vi "setUp.vi"(8 "error in (no error)":errorcluster, 11 "reference in":refnum<class "RT Stop.lvclass">) -> (0 "error out":errorcluster, 3 "reference out":refnum<class "RT Stop.lvclass">)   [LabVIEW 2016, in "RT Stop.lvclass"]
doc: "setUp runs prior to the test method during test execution. Use this method to initialize any object data required by your tests."
uses:
  RT Stop.lvclass
  D:/Programs/National Instruments/LabVIEW 2016/vi.lib/addons/_JKI Toolkits/VI Tester/TestCase.llb/TestCase.lvclass
  RT Stop.lvclass/RT Stop.ctl
  <vilib>/addons/_JKI Toolkits/VI Tester/TestCase.llb/TestCase.lvclass
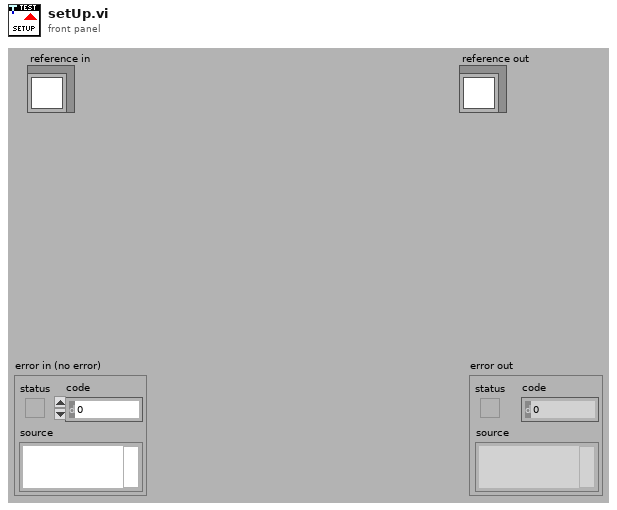
[diagram p1: front panel]
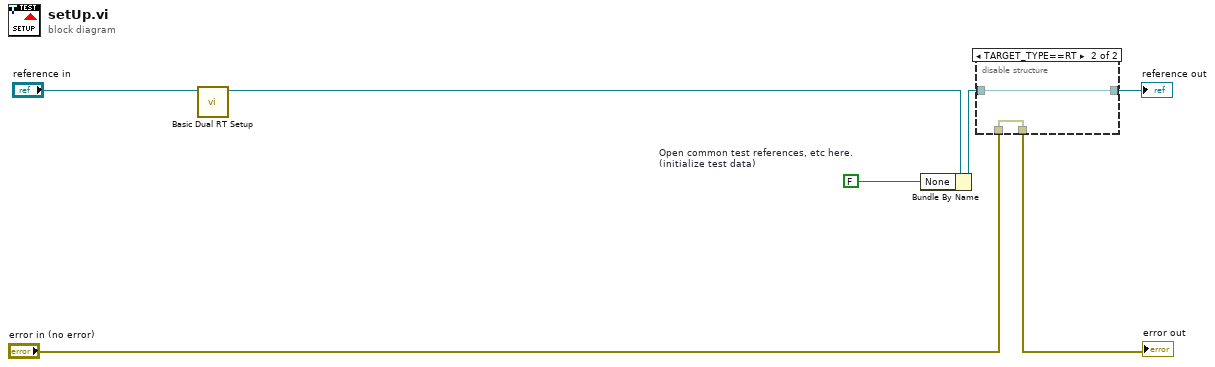
[diagram p0: block diagram]
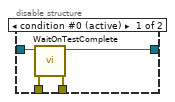
[diagram p2: hidden frame]
diagram:
  w3 = FALSE  # Open common test references, etc here. (initialize test data)
  n1 = call-dynamic "Basic Dual RT Setup.vi"("1553 Test in"="reference in") -> ("1553 Test out"=w1:refnum<class "RT Stop.lvclass">)  [unwired: 9 in, 1 out]
  n2 = Bundle By Name(cluster=w1, "None"=w3) -> (w4:refnum<class "RT Stop.lvclass">)
  n3 = disable-structure shown="TARGET_TYPE==RT" {
    disable-tunnel: "error in (no error)" -> [w11 w12]
    disable-tunnel: [w10 w12] -> w6
    disable-tunnel: [w9 w13] -> w5
    disable-tunnel: w4 -> [w8 w13]
    frame condition #0 (active) {
      n4 = call <vilib>:"WaitOnTestComplete.vi"("error in (no error)"=w11, "TestCase in"=w8) -> ("error out"=w10:errorcluster, "TestCase out"=w9:refnum<class "RT Stop.lvclass">)  [unwired: 8 in]
    }
    frame condition #1 {
    }
  }
  "error out" <- w6
  "reference out" <- w5
